vi "Упр. видимостью мишеней (SubVI).vi"(2 "Строка параметров видимости мишеней":string, 7 "Кластер reference":T1) -> (3 "Кластер reference out":T1, 13 "Остаток строки":string, 15 "Кол-во видимых мишеней":u8)   [LabVIEW 2013]
doc: "Включение видимости мишеней"
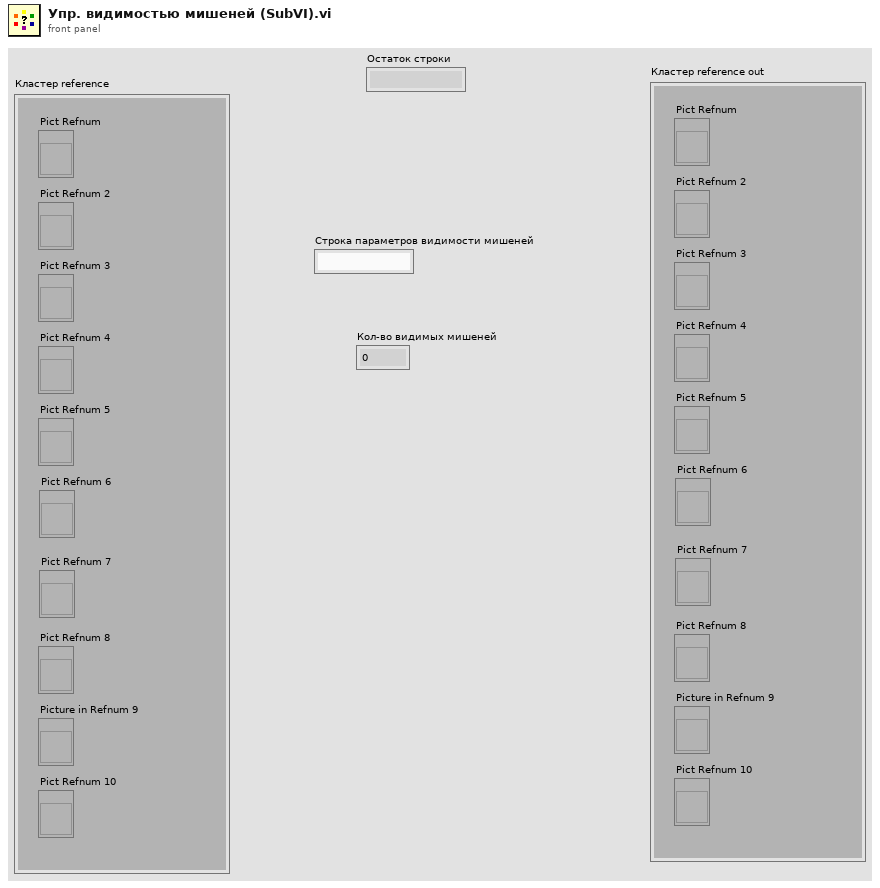
[diagram p1: front panel]
types:
  T1 = cluster{"Pict Refnum":refnum<vi>, "Pict Refnum 2":refnum<vi>, "Pict Refnum 3":refnum<vi>, "Pict Refnum 4":refnum<vi>, "Pict Refnum 5":refnum<vi>, "Pict Refnum 6":refnum<vi>, "Pict Refnum 7":refnum<vi>, "Pict Refnum 8":refnum<vi>, "Picture in Refnum 9":refnum<vi>, "Pict Refnum 10":refnum<vi>}
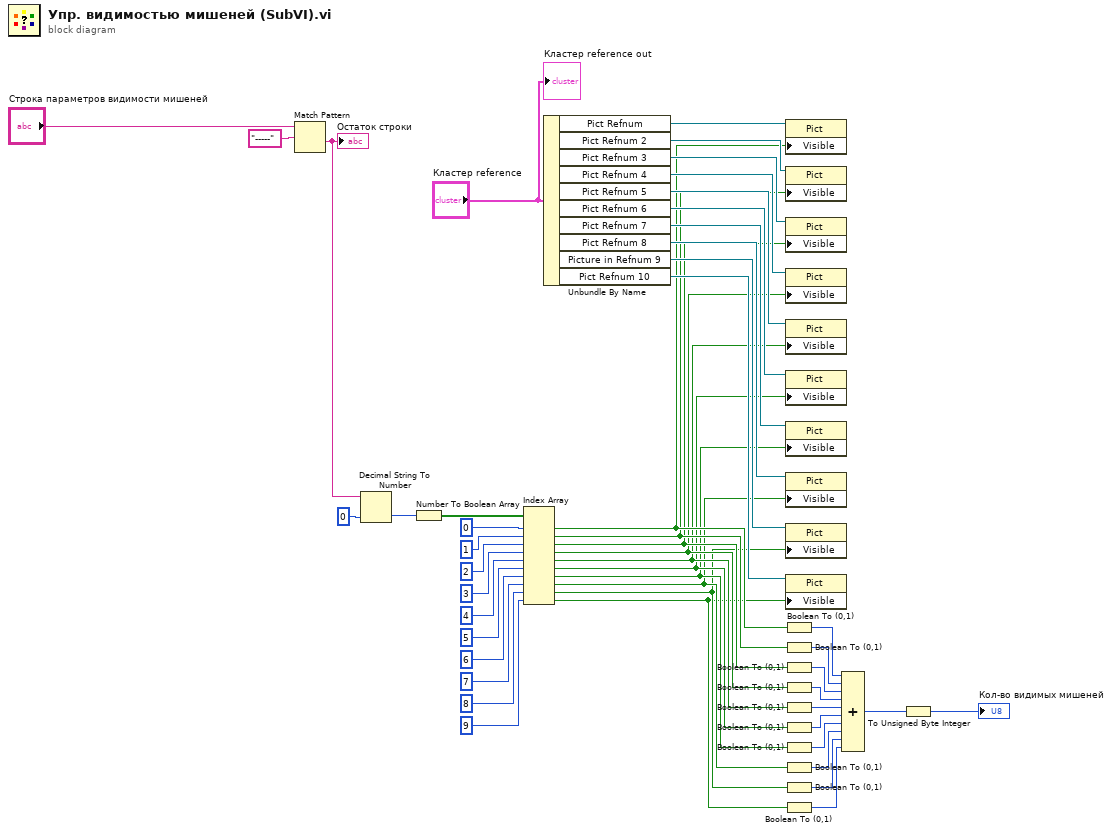
[diagram p0: block diagram]
diagram:
  n1 = Match Pattern(string="Строка параметров видимости мишеней", regular expression="-----") -> (after substring=w24:string)  [unwired: 1 in, 3 out]
  "Остаток строки" <- w24
  n2 = Decimal String To Number(string=w24, default (0L)=u16 0 ("default (0 I32)")) -> (number=w29:u16)  [unwired: 1 in, 1 out]
  n3 = Number To Boolean Array(number=w29) -> (Boolean array=w26:bool[])
  n4 = Index Array(array=w26, index #1=0 ("index"), index #2=1 ("index"), index #3=2 ("index"), index #4=3 ("index"), index #5=4 ("index"), index #6=5 ("index"), index #7=6 ("index"), index #8=7 ("index"), index #9=8 ("index"), index #10=9 ("index")) -> (element #1=w22:bool, element #2=w21:bool, element #3=w20:bool, element #4=w19:bool, element #5=w18:bool, element #6=w17:bool, element #7=w16:bool, element #8=w15:bool, element #9=w14:bool, element #10=w13:bool)
  n5 = Unbundle By Name("Кластер reference") -> ("Pict Refnum"=w39:refnum<vi>, "Pict Refnum 2"=w38:refnum<vi>, "Pict Refnum 3"=w37:refnum<vi>, "Pict Refnum 4"=w36:refnum<vi>, "Pict Refnum 5"=w35:refnum<vi>, "Pict Refnum 6"=w34:refnum<vi>, "Pict Refnum 7"=w33:refnum<vi>, "Pict Refnum 8"=w32:refnum<vi>, "Picture in Refnum 9"=w31:refnum<vi>, "Pict Refnum 10"=w30:refnum<vi>)
  n6 = Boolean To (0,1)(Boolean=w22) -> (0, 1=w12:i16)
  n7 = Boolean To (0,1)(Boolean=w21) -> (0, 1=w11:i16)
  n8 = Boolean To (0,1)(Boolean=w20) -> (0, 1=w10:i16)
  n9 = Boolean To (0,1)(Boolean=w19) -> (0, 1=w9:i16)
  n10 = Boolean To (0,1)(Boolean=w18) -> (0, 1=w8:i16)
  n11 = Boolean To (0,1)(Boolean=w17) -> (0, 1=w7:i16)
  n12 = Boolean To (0,1)(Boolean=w16) -> (0, 1=w6:i16)
  n13 = Boolean To (0,1)(Boolean=w15) -> (0, 1=w5:i16)
  n14 = Boolean To (0,1)(Boolean=w14) -> (0, 1=w4:i16)
  n15 = Boolean To (0,1)(Boolean=w13) -> (0, 1=w3:i16)
  n16 = property on="Property Node" class="Pict"(reference=w39, "Visible"=w22) -> ()  [unwired: 1 in, 2 out]
  n17 = property on="Property Node" class="Pict"(reference=w38, "Visible"=w21) -> ()  [unwired: 1 in, 2 out]
  n18 = property on="Property Node" class="Pict"(reference=w37, "Visible"=w20) -> ()  [unwired: 1 in, 2 out]
  n19 = property on="Property Node" class="Pict"(reference=w36, "Visible"=w19) -> ()  [unwired: 1 in, 2 out]
  n20 = property on="Property Node" class="Pict"(reference=w35, "Visible"=w18) -> ()  [unwired: 1 in, 2 out]
  n21 = property on="Property Node" class="Pict"(reference=w34, "Visible"=w17) -> ()  [unwired: 1 in, 2 out]
  n22 = property on="Property Node" class="Pict"(reference=w33, "Visible"=w16) -> ()  [unwired: 1 in, 2 out]
  n23 = property on="Property Node" class="Pict"(reference=w32, "Visible"=w15) -> ()  [unwired: 1 in, 2 out]
  n24 = property on="Property Node" class="Pict"(reference=w31, "Visible"=w14) -> ()  [unwired: 1 in, 2 out]
  n25 = property on="Property Node" class="Pict"(reference=w30, "Visible"=w13) -> ()  [unwired: 1 in, 2 out]
  n26 = Compound Arithmetic op=ADD(w12, w11, w10, w9, w8, w7, w6, w5, w4, w3) -> (w2:i16)
  n27 = To Unsigned Byte Integer(number=w2) -> (unsigned 8bit integer=→"Кол-во видимых мишеней":u8)
  "Кластер reference out" <- "Кластер reference"
